vi "Controller_Main.vi"(8 "error in (no error)":errorcluster) -> (0 "error out":errorcluster)   [LabVIEW 2017]
doc: "This is Top Level VI for Controller Module. You can communicate with this module using its API. Communication is made based on queue. This module has not User Interface so I chase State Machine architecture."
uses:
  General/Controls/#TD_General_CommunicationQueueStates_Enum.ctl
  Private controls/#TD_Controller_InnerData_Cluster.ctl
  Private controls/#TD_Controller_ModuleStates_Enum.ctl
  Private controls/#TD_Controller_ModuleData_Cluster.ctl
  General/Controls/#TD_General_FromWho_Enum.ctl
  Private controls/#TD_Controller_CurrentOperation.ctl
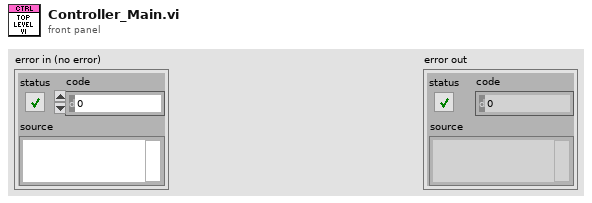
[diagram p1: front panel]
types:
  T1 = typedef "#TD_General_CommunicationQueueStates_Enum.ctl" = enum16{"ERROR_Default", "Obtain", "GetRef", "Enqueue", "EnqueueAtOpp", "GetStatus", "Release"}
  T2 = typedef "#TD_General_FromWho_Enum.ctl" = enum16{"ERROR_Default", "UserConsole", "DisplayConsole", "SensorInterface", "Controller", "Database", "Timing", "AdditionalModule", "ErrorHandling"}
  T3 = typedef "#TD_Controller_ModuleStates_Enum.ctl" = enum16{"ERROR_Default", "Init", "Close", "ErrorHandling", "NumberKeyPressed", "CKeyPressed", "EKeyPressed", "TransPressed", "CardReadPressed", "DepositPressed", "FundsPressed", "TimeElapsed", "DB_Responds", "ExecuteIdle"}
  T4 = typedef "#TD_Controller_ModuleData_Cluster.ctl" = cluster{"Action":T3, "Data":variant}
  T5 = typedef "#TD_General_IntermoduleData_Cluster.ctl" = cluster{"Sender":T2, "ModuleData":variant}
  T6 = typedef "#TD_Controller_InnerData_Cluster.ctl" = cluster{"Sth":bool, "CurrentOperation":T7, "Attemps":i32}
  T7 = typedef "#TD_Controller_CurrentOperation.ctl" = enum16{"ERROR_Default", "Init", "Login", "Idle", "Balance", "FastCash", "Deposit", "Withdrawal"}
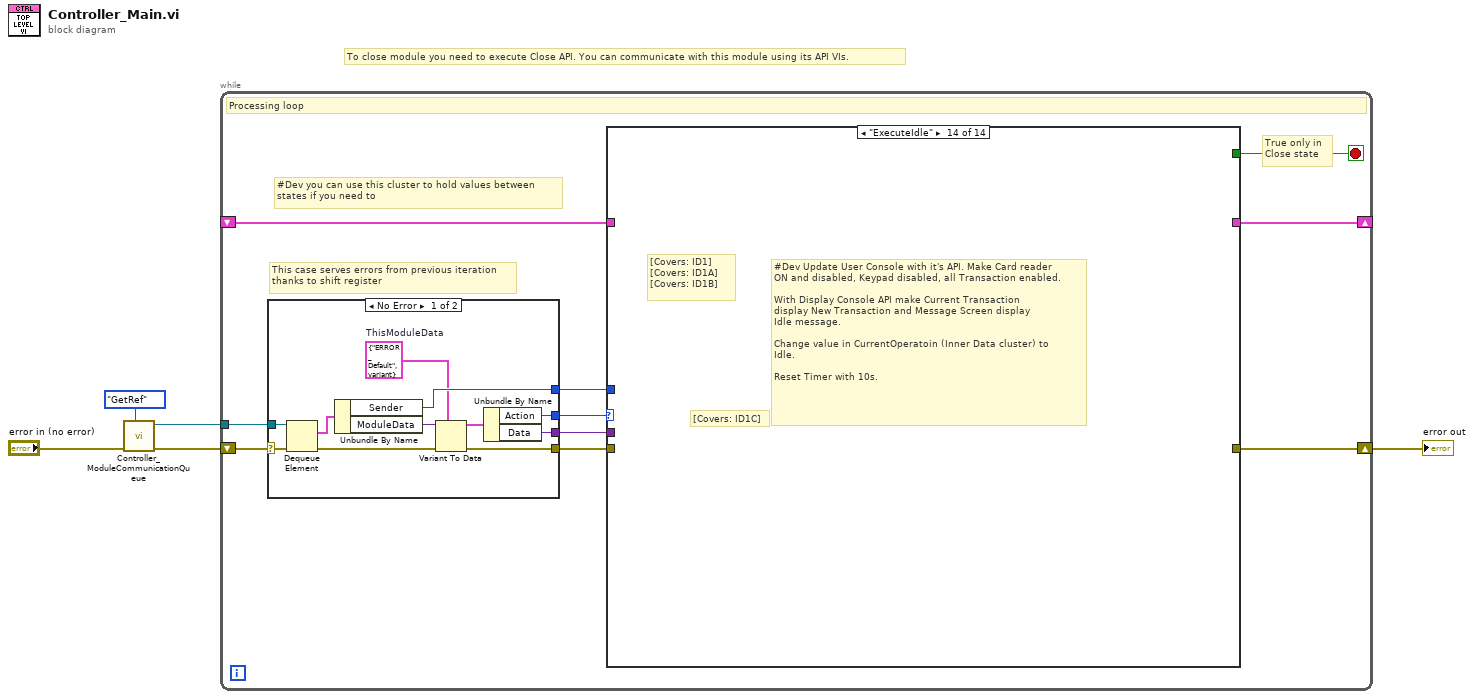
[diagram p0: block diagram]
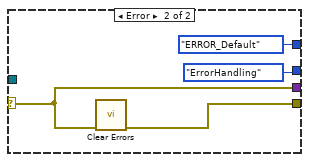
[diagram p2: hidden frame]
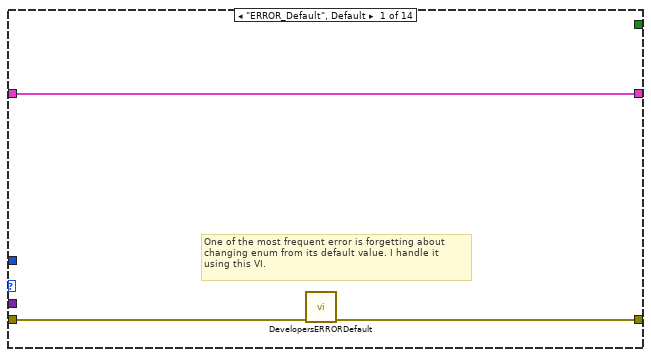
[diagram p3: hidden frame]
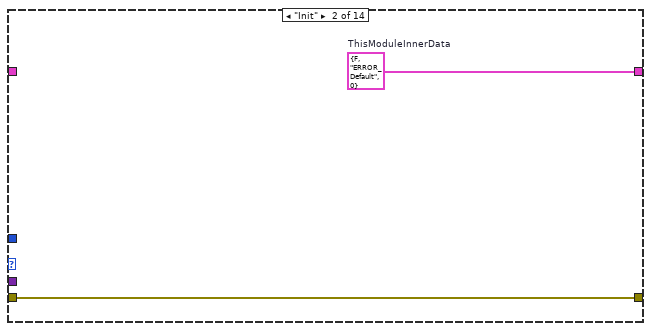
[diagram p4: hidden frame]
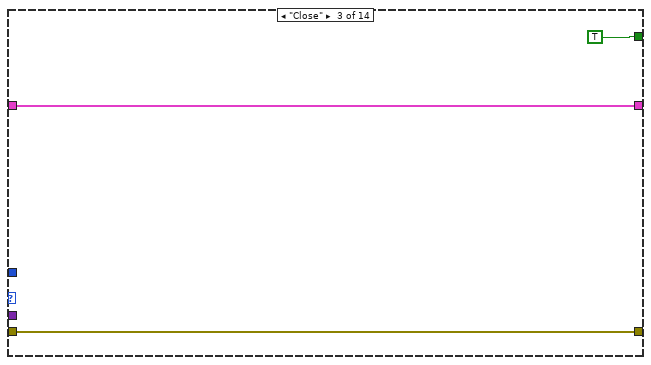
[diagram p5: hidden frame]
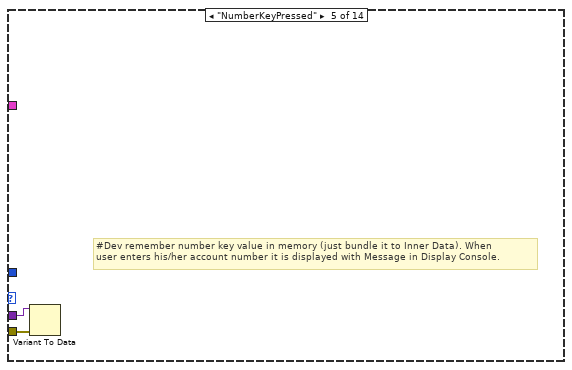
[diagram p7: hidden frame]
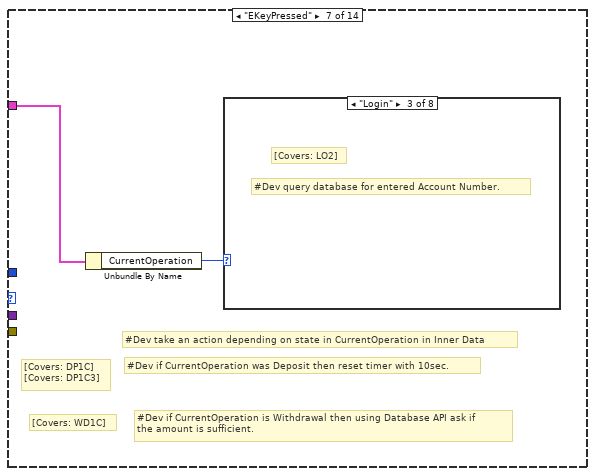
[diagram p9: hidden frame]
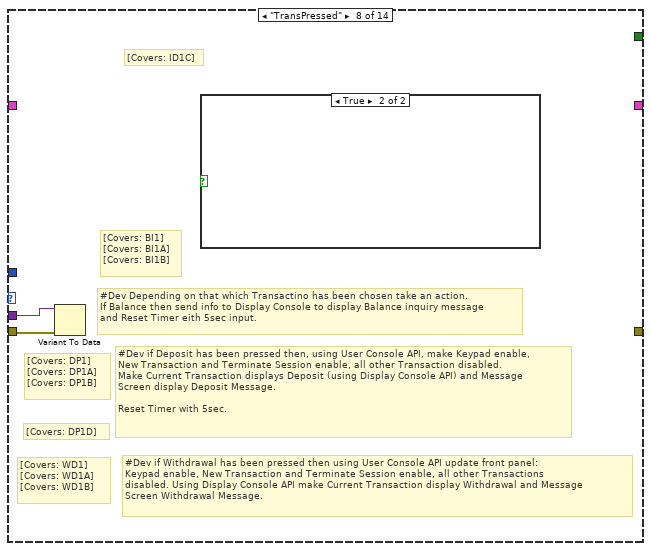
[diagram p17: hidden frame]
diagram:
  # "To close module you need to execute Close API. You can communicate with this module using its API VIs."
  n1 = call "Controller_ModuleCommunicationQueue.vi"("Action"=#TD_General_CommunicationQueueStates_Enum."GetRef", "error in (no error)"="error in (no error)") -> ("error out"=w2:errorcluster, "Ref out"=w3:refnum<queue>)  [unwired: 7 in, 1 out]
  n2 = while {
    tunnel: w3 -> [w14]
    shift-right: [w7] -> w1
    shift-left: w2 -> [w15]
    shift-right: [w13] -> _
    shift-left: _ -> [w12]
    stop <- w6 stop-if-true
    # "True only in \nClose state"
    # "#Dev you can use this cluster to hold values between \nstates if you need to"
    # "This case serves errors from previous iteration \nthanks to shift register"
    # "Processing loop"
    n3 = case shown="No Error" w15 {
      selector: w15 -> [w26 w30]
      tunnel: w14 -> [w25 _]
      tunnel: [w21 #TD_General_FromWho_Enum."ERROR_Default" ("Sender")] -> w11
      tunnel: [w18 #TD_Controller_ModuleStates_Enum."ErrorHandling" ("Action")] -> w10
      tunnel: [w17 w30] -> w9
      tunnel: [w16 w29] -> w8
      frame No Error {
        w20 = T4 {"Action"=enum."ERROR_Default", "Data"=variant}  # ThisModuleData
        n4 = Dequeue Element(queue=w25, error in (no error)=w26) -> (element=w24:T5, error out=w22:errorcluster)  [unwired: 1 in, 2 out]
        n5 = Unbundle By Name(w24) -> ("Sender"=w21:T2, "ModuleData"=w23:variant)
        n6 = Variant To Data(error in=w22, type=w20, Variant=w23) -> (data=w19:T4, error out=w16:errorcluster)
        n7 = Unbundle By Name(w19) -> ("Action"=w18:T3, "Data"=w17:variant)
      }
      frame Error {
        n8 = call <vilib>:"Clear Errors.vi"("error in (no error)"=w30) -> ("error out"=w29:errorcluster)  [unwired: 5 in, 1 out]
      }
    }
    n9 = case shown="\"ExecuteIdle\"" w10 {
      tunnel: [w33 w35 w37 w40 _ _ _ _ _ _ _ _ _ _] -> w13
      tunnel: w12 -> [w33 _ w37 w40 _ _ w44 _ _ _ _ _ _ _]
      tunnel: w11 -> [_ _ _ _ _ _ _ _ _ _ _ _ _ _]
      tunnel: w9 -> [_ _ _ _ w42 _ _ w45 _ _ _ _ _ _]
      tunnel: w8 -> [w32 w34 w36 w39 w41 _ _ w46 _ _ _ _ _ _]
      tunnel: [w31 w34 w36 w39 _ _ _ _ _ _ _ _ _ _] -> w7
      tunnel: [_ _ TRUE _ _ _ _ _ _ _ _ _ _ _] -> w6
      frame "ERROR_Default", Default {
        # "One of the most frequent error is forgetting about \nchanging enum from its default value. I handle it \nusing this VI."
        n10 = call "DevelopersERRORDefault.vi"("error in (no error)"=w32) -> ("error out"=w31:errorcluster)  [unwired: 10 in]
      }
      frame "Init" {
        w35 = T6 {"Sth"=FALSE, "CurrentOperation"=enum."ERROR_Default", "Attemps"=0}  # ThisModuleInnerData
      }
      frame "Close" {
      }
      frame "ErrorHandling" {
        # "#Dev take some actions to handle the error \nand inform central Error Handling Module \nabout this error using Error Handling Module \nAPI"
      }
      frame "NumberKeyPressed" {
        # "#Dev remember number key value in memory (just bundle it to Inner Data). When \nuser enters his/her account number it is displayed with Message in Display Console."
        n11 = Variant To Data(error in=w41, Variant=w42) -> ()  [unwired: 1 in, 2 out]
      }
      frame "CKeyPressed" {
        # "#Dev clear what was entered in NumberKeyPressed state"
      }
      frame "EKeyPressed" {
        # "[Covers: WD1C]"
        # "#Dev if CurrentOperation is Withdrawal then using Database API ask if \nthe amount is sufficient."
        # "[Covers: DP1C]  \n[Covers: DP1C3]"
        # "#Dev if CurrentOperation was Deposit then reset timer with 10sec."
        # "#Dev take an action depending on state in CurrentOperation in Inner Data"
        n12 = Unbundle By Name(w44) -> ("CurrentOperation"=w43:T7)
        n13 = case shown="\"Login\"" w43 {
          frame "ERROR_Default", Default {
          }
          frame "Init" {
          }
          frame "Login" {
            # "#Dev query database for entered Account Number."
            # "[Covers: LO2]"
          }
          frame "Idle" {
          }
          frame "Balance" {
          }
          frame "FastCash" {
          }
          frame "Deposit" {
          }
          frame "Withdrawal" {
          }
        }
      }
      frame "TransPressed" {
        # "[Covers: WD1] \n[Covers: WD1A]  \n[Covers: WD1B]"
        # "#Dev if Withdrawal has been pressed then using User Console API update front panel: \nKeypad enable, New Transaction and Terminate Session enable, all other Transactions \ndisabled. Using Display Console API make Current Transaction display Withdrawal and Message \nScreen Withdrawal Message."
        # "[Covers: DP1D]"
        # "[Covers: DP1] \n[Covers: DP1A] \n[Covers: DP1B]"
        # "#Dev if Deposit has been pressed then, using User Console API, make Keypad enable, \nNew Transaction and Terminate Session enable, all other Transaction disabled. \nMake Current Transaction displays Deposit (using Display Console API) and Message \nScreen display Deposit Message.\n\nReset Timer with 5sec."
        # "[Covers: ID1C]"
        # "[Covers: BI1] \n[Covers: BI1A] \n[Covers: BI1B]"
        # "#Dev Depending on that which Transactino has been chosen take an action. \nIf Balance then send info to Display Console to display Balance inquiry message \nand Reset Timer eith 5sec input."
        n14 = Variant To Data(error in=w46, Variant=w45) -> ()  [unwired: 1 in, 2 out]
        n15 = case shown="True" {
          selector: _ -> [_ _]
          frame False {
          }
          frame True {
          }
        }
      }
      frame "CardReadPressed" {
        # "[Covers: LO1] \n[Covers: LO1B]\n[Covers: LO2]\n[Covers: LO2A]"
        # "#Dev Update front panel of User Console and Display console \nusing its API. Change CurrentOperation enum (Inner Data cluster) \nto Login. Reset Timer_01 with 10 seconds."
      }
      frame "DepositPressed" {
        # "#Dev using Database API update balance"
        # "[Covers: DP1C2]"
      }
      frame "FundsPressed" {
        # "[Covers: WD1D]"
        # "#Dev return to Idle state"
      }
      frame "TimeElapsed" {
        # "[Covers: WD1E]"
        # "#Dev If CurrentOperation was withdrawal and there \nare no sufficient funds then execute Idle State."
        # "#Dev go to Terminate state if CurrentOperation was Deposit"
        # "[Covers: DP1C1]"
        # "[Covers: LO2A]"
        # "Unbundle CurrentOperation and based on that decide what action \nto take."
      }
      frame "DB_Responds" {
        # "[Covers: WD1D]"
        # "#Dev if Database was responding to question about sufficient amount then \nsend to Dislay Console (using it's API) info about Withdrawal Complete. \nReset Timer.\n\nIf there are no sufficient funds then send to Display Console info about \nfail and also Reset Timer."
        # "[Covers: LO3] \n[Covers: LO3A] \n[Covers: LO3B] \n[Covers: LO3C] \n[Covers: LO3C1] \n[Covers: LO3C2]"
        # "#Dev read from Variant data to which query DataBase has responded and execute \napriopriate case in case structure.  \n\nBased on that ex. execute Idle stat if the Account Number is found. If user enters an \nincorrect Account Number send info about it to Display Console to update the message. \nCount login attempts (store info about attempts in Inner Data)"
      }
      frame "ExecuteIdle" {
        # "[Covers: ID1C]"
        # "#Dev Update User Console with it's API. Make Card reader \nON and disabled, Keypad disabled, all Transaction enabled.\n \nWith Display Console API make Current Transaction \ndisplay New Transaction and Message Screen display \nIdle message. \n\nChange value in CurrentOperatoin (Inner Data cluster) to \nIdle.\n\nReset Timer with 10s."
        # "[Covers: ID1] \n[Covers: ID1A]   \n[Covers: ID1B]"
      }
    }
  }
  "error out" <- w1
